vi "PositionReceiverAngleGoal.vi"(8 "error in (no error)":errorcluster, 9 "atacando contra":bool, 10 "Game":refnum<class "Game.lvclass">, 11 "PositionToReceivePassSkill in":refnum<class "PositionToReceivePassSkill.lvclass">) -> (0 "error out":errorcluster, 2 "theta final":dbl, 3 "PositionToReceivePassSkill out":refnum<class "PositionToReceivePassSkill.lvclass">)   [LabVIEW 2023, in "PositionToReceivePassSkill.lvclass"]
uses:
  PositionToReceivePassSkill.lvclass
  Game_class/Game.lvclass
  Game_class/Game.lvclass/Game.ctl
  Object_class/Object.lvclass/Object.ctl
  Team_class/Team.lvclass/Team.ctl
  Robot_class/roles.ctl
  Robot_class/Robot.lvclass/Robot.ctl
  Object_class/Read x.vi
  Object_class/Write x.vi
  Robot_class/Read role.vi
  Robot_class/Read id.vi
  Object_class/Read y.vi
  Game_class/Read BallRef.vi
  Game_class/Read EnemyRef.vi
  Game_class/Read FieldRef.vi
  Game_class/Read DefensiveTeam.vi
  Game_class/Read KeeperTeam.vi
  Team_class/Read RobotRef.vi
  Ally_class/Ally.lvclass
  Enemy_class/Enemy.lvclass
  Robot_class/Robot.lvclass
  Ball_class/Ball.lvclass
  Field_class/Field.lvclass
panel:
  in  "Array":dbl[](array[numeric])=[0.0, 0.0, 0.0, 0.0, 0.0, 0.0]
  in  "Contador 2":dbl
  in  "fim do intervalo":dbl=-1.57
  in  "inicio do intervalo":dbl=-1.57
  in  "tamanho do intervalo":dbl
  in  "valor de theta":dbl
  in  "RobôsParaAnalisar":dbl[][](array[numeric])=[[99999.0, 99999.0], [99999.0, 99999.0], [99999.0, 99999.0], [99999.0, 99999.0], [99999.0, 99999.0], [99999.0, 99999.0], [99999.0, 99999.0]]
  in  "Contador":dbl
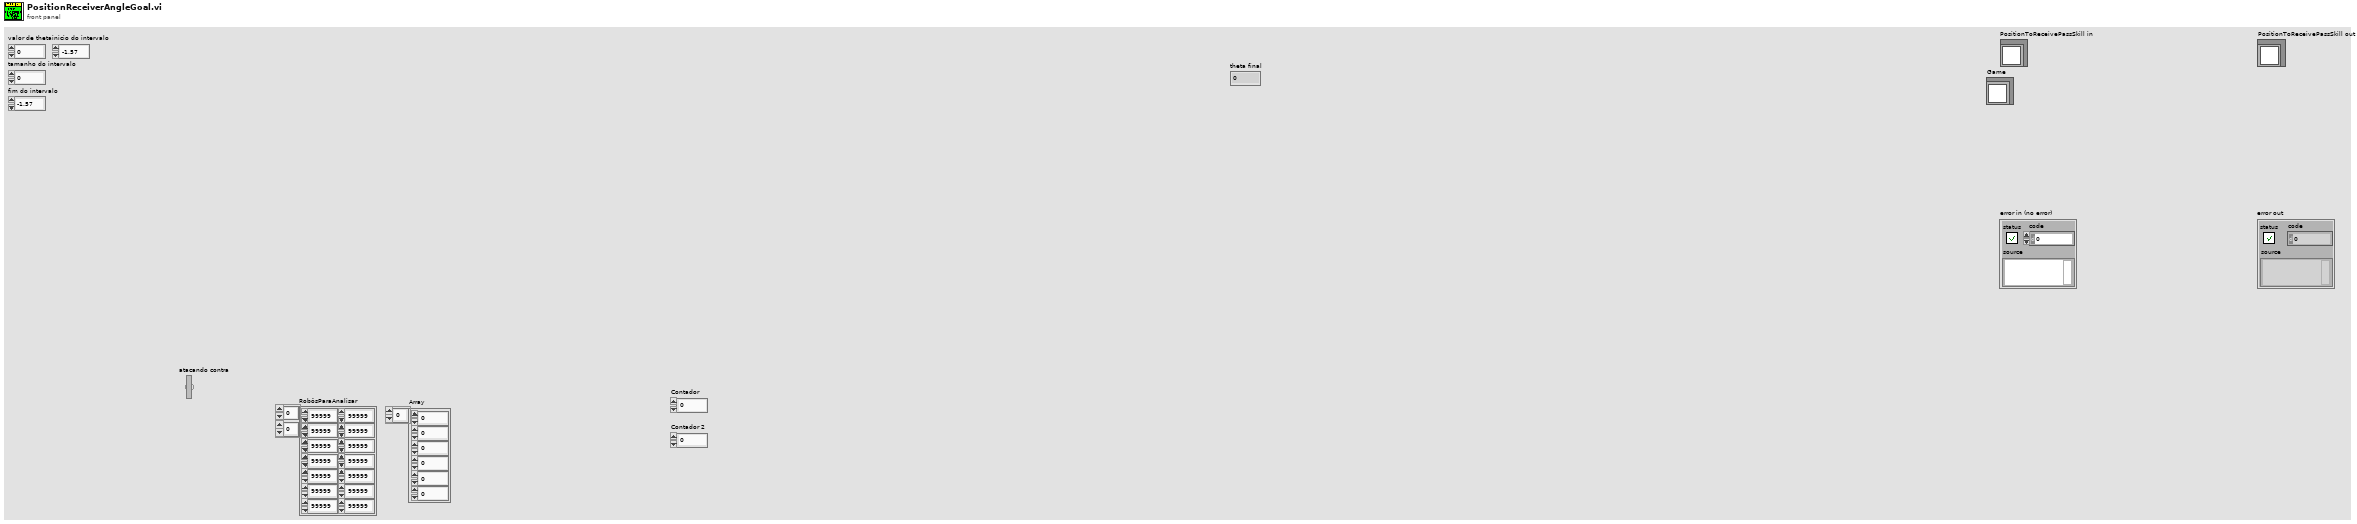
[diagram p1: front panel]
types:
  T1 = typedef "roles.ctl" = enum16{"BallChallengerAttackerVSS", "NormalAttackerVSS", "AttackerAimGoalVSS", "DefenderAreaVSS", "KeeperVSS", "Tabler", "TableFinalizer", "PrepareRollToPassRoller", "PrepareRollToPassReceiver", "SimplePassRoll", "SimplePassRollReceiver", "PenaltyDefense", "PreparePassReceiver 2", "PreparePassReceiver 1", "PassObserver", "Timeout", "Goto", "ZigZag", "None", "BallOutOfField", "DefenderArea", "Duelist", "AttackerStop", "FollowAttacker", "KeeperRole", "KickPenalty", "AttackerAimGoal", "AttackerBlock", "Marker", "Halt", "Shoot", "PassKicker", "PassReceiver", "TestRole", "PenaltyAttacker"}
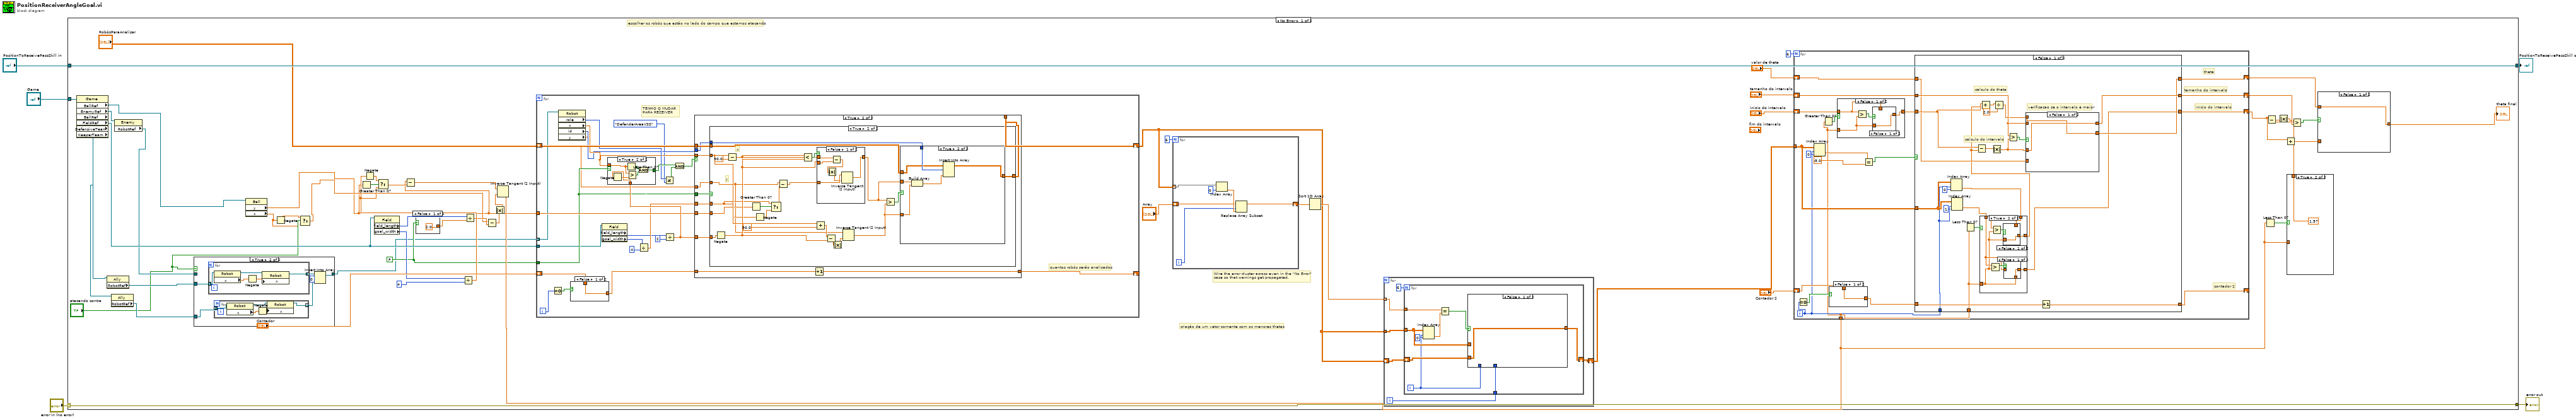
[diagram p0: block diagram]
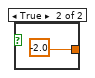
[diagram p4: hidden frame]
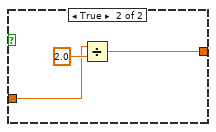
[diagram p5: hidden frame]
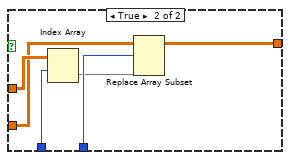
[diagram p6: hidden frame]
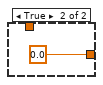
[diagram p9: hidden frame]
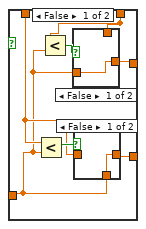
[diagram p10: hidden frame]
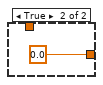
[diagram p17: hidden frame]
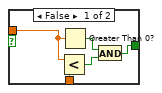
[diagram p18: hidden frame]
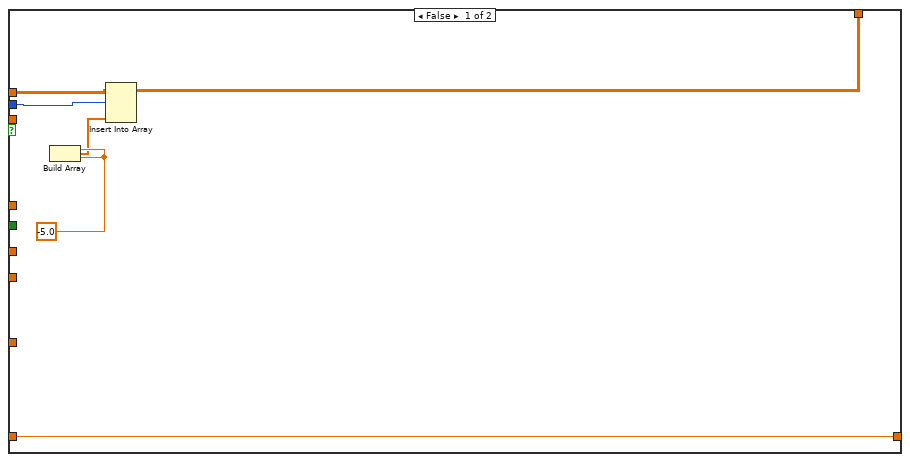
[diagram p19: hidden frame]
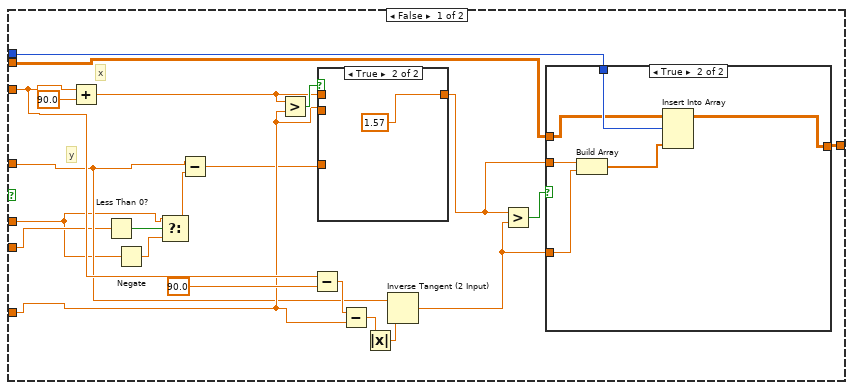
[diagram p20: hidden frame]
diagram:
  n1 = case shown="No Error" "error in (no error)" {
    selector: "error in (no error)" -> [w58 w333]
    tunnel: [w58 w333] -> w4
    tunnel: [w59 w332] -> w2
    tunnel: "PositionToReceivePassSkill in" -> [w59 w332]
    tunnel: "Game" -> [w23 _]
    frame No Error {
      w18 = FALSE
      # "criação de um vetor somente com os menores thetas"
      # "escolher os robôs que estão no lado do campo que estamos atacando"
      # "Wire the error cluster across even in the \"No Error\"\ncase so that warnings get propagated."
      n2 = property class="Game" props=["BallRef", "EnemyRef", "BallRef", "FieldRef", "DefensiveTeam", "KeeperTeam"](reference=w23) -> ("BallRef"=w9:refnum<class "Ball.lvclass">, "EnemyRef"=w22:refnum<class "Enemy.lvclass">, "FieldRef"=w21:refnum<class "Field.lvclass">, "DefensiveTeam"=w16:refnum<class "Ally.lvclass">, "KeeperTeam"=w11:refnum<class "Ally.lvclass">)  [unwired: 1 in, 3 out]
      n3 = property class="Ally"(reference=w16) -> ("RobotRef"=w14:refnum<class "Robot.lvclass">[])  [unwired: 1 in, 2 out]
      n4 = property class="Ally"(reference=w11) -> ("RobotRef"=w12:refnum<class "Robot.lvclass">[])  [unwired: 1 in, 2 out]
      n5 = property class="Enemy"(reference=w22) -> ("RobotRef"=w15:refnum<class "Robot.lvclass">[])  [unwired: 1 in, 2 out]
      n6 = case shown="True" "atacando contra" {
        tunnel: [w60 w61] -> w13
        tunnel: w15 -> [w60 _]
        tunnel: w14 -> [_ w66]
        tunnel: w12 -> [_ w65]
        frame False {
        }
        frame True {
          n7 = for {
            tunnel: [w74] -> w64 mode=indexing
            tunnel: w66 -> [w72] mode=indexing
            n8 = property class="Robot"(reference=w72) -> (reference out=w73:refnum<class "Robot.lvclass">, "x"=w76:dbl)  [unwired: 1 in, 1 out]
            n9 = Negate(x=w76) -> (-x=w75:dbl)
            n10 = property class="Robot"(reference=w73, "x"=w75) -> (reference out=w74:refnum<class "Robot.lvclass">)  [unwired: 1 in, 1 out]
          }
          n11 = for {
            tunnel: w65 -> [w71] mode=indexing
            tunnel: [w67] -> w63 mode=indexing
            n12 = property class="Robot"(reference=w71) -> (reference out=w68:refnum<class "Robot.lvclass">, "x"=w70:dbl)  [unwired: 1 in, 1 out]
            n13 = Negate(x=w70) -> (-x=w69:dbl)
            n14 = property class="Robot"(reference=w68, "x"=w69) -> (reference out=w67:refnum<class "Robot.lvclass">)  [unwired: 1 in, 1 out]
          }
          n15 = Insert Into Array(array=w64, index=0, new element=w63) -> (w61:refnum<class "Robot.lvclass">[])
        }
      }
      n16 = property class="Ball"(reference=w9) -> ("y"=w7:dbl, "x"=w6:dbl)  [unwired: 1 in, 2 out]
      n17 = Negate(x=w6) -> (-x=w8:dbl)
      n18 = Select(t=w8, s="atacando contra", f=w6) -> (s? t:f=w30:dbl)
      n19 = Greater Than 0?(x=w7) -> (x > 0?=w35:bool)
      n20 = property class="Field"(reference=w21) -> ("field_length"=w20:i32, "goal_width"=w19:i32)  [unwired: 1 in, 2 out]
      n21 = case shown="False" w18 {
        tunnel: [2.0 ("y") -2.0 ("y")] -> w28
        frame False {
        }
        frame True {
        }
      }
      n22 = Divide(x=w19, y=u32 4) -> (x/y=w33:dbl)
      n23 = Negate(x=w33) -> (-x=w34:dbl)
      n24 = Select(t=w34, s=w35, f=w33) -> (s? t:f=w32:dbl)
      n25 = Subtract(x=w7, y=w32) -> (x-y=w29:dbl)
      n26 = Divide(x=w20, y=w28) -> (x/y=w31:dbl)
      n27 = Subtract(x=w30, y=w31) -> (x-y=w25:dbl)
      n28 = Absolute Value(x=w25) -> (abs(x)=w24:dbl)
      n29 = Inverse Tangent (2 Input)(1:w24, 2:w29) -> (0:w26:dbl)
      n30 = for {
        tunnel: w13 -> [w202] mode=indexing
        tunnel: w18 -> [w207]
        shift-right: [w212] -> w46
        shift-left: "RobôsParaAnalisar" -> [w218]
        shift-right: [w213] -> _
        shift-left: "Contador" -> [w215]
        tunnel: w21 -> [w197]
        tunnel: w7 -> [w210]
        i -> [w216]
        # "TENHO Q MUDAR \nPARA RECEIVER"
        # "quantos robôs serão analisados"
        n31 = Equal To 0?(x=w216) -> (x = 0?=w217:bool)
        n32 = property class="Robot"(reference=w202) -> ("role"=w201:T1, "x"=w200:dbl, "id"=w199:i32, "y"=w198:dbl)  [unwired: 1 in, 2 out]
        n33 = case shown="False" w217 {
          tunnel: w215 -> [w219 _]
          tunnel: [w219 0.0] -> w214
          frame False {
          }
          frame True {
          }
        }
        n34 = property class="Field"(reference=w197) -> ("field_length"=w196:i32, "goal_width"=w195:i32)  [unwired: 1 in, 2 out]
        n35 = Divide(x=w195, y=u32 4) -> (x/y=w208:dbl)
        n36 = Not Equal?(x=w201, y=roles."DefenderAreaVSS") -> (x != y?=w204:bool)
        n37 = Divide(x=w196, y=u32 2) -> (x/y=w211:dbl)
        n38 = case shown="True" w207 {
          tunnel: w200 -> [w225 w226]
          tunnel: [w221 w231] -> w203
          tunnel: w211 -> [w224 w227]
          frame False {
            n39 = Less?(x=w225, y=w224) -> (x < y?=w222:bool)
            n40 = Greater Than 0?(x=w225) -> (x > 0?=w223:bool)
            n41 = And(x=w223, y=w222) -> (x .and. y?=w221:bool)
          }
          frame True {
            n42 = Negate(x=w227) -> (-x=w228:dbl)
            n43 = Less Than 0?(x=w226) -> (x < 0?=w230:bool)
            n44 = Greater?(x=w226, y=w228) -> (0:w229:bool)
            n45 = And(x=w230, y=w229) -> (x .and. y?=w231:bool)
          }
        }
        n46 = And(x=w203, y=w204) -> (x .and. y?=w205:bool)
        n47 = case shown="True" w205 {
          tunnel: w218 -> [w236 w243]
          tunnel: w199 -> [w235 w241]
          tunnel: w200 -> [_ w245]
          tunnel: w198 -> [_ w242]
          tunnel: w214 -> [w237 w247]
          tunnel: [w237 w248] -> w213
          tunnel: [w232 w240] -> w212
          tunnel: w207 -> [_ w246]
          tunnel: w211 -> [_ w244]
          tunnel: w210 -> [_ w239]
          tunnel: w208 -> [_ w238]
          frame False {
            w234 = -5.0 ("element")
            n48 = Build Array(w234, w234) -> (w233:dbl[])
            n49 = Insert Into Array(array=w236, index (row)=w235, new element=w233) -> (w232:dbl[][])  [unwired: 1 in]
          }
          frame True {
            n50 = case shown="True" w246 {
              tunnel: w245 -> [w260 w308]
              tunnel: w244 -> [w259 w311]
              tunnel: w243 -> [w261 w303]
              tunnel: w242 -> [w252 w292]
              tunnel: w241 -> [w262 w302]
              tunnel: [w258 w299] -> w240
              tunnel: w239 -> [w251 w296]
              tunnel: w238 -> [w250 w293]
              frame False {
                # "y"
                # "x"
                n51 = Add(x=w260, y=90.0) -> (x+y=w268:dbl)
                n52 = Less Than 0?(x=w251) -> (x < 0?=w255:bool)
                n53 = Negate(x=w250) -> (-x=w254:dbl)
                n54 = Select(t=w250, s=w255, f=w254) -> (s? t:f=w253:dbl)
                n55 = Subtract(x=w252, y=w253) -> (x-y=w249:dbl)
                n56 = Greater?(x=w268, y=w259) -> (0:w269:bool)
                n57 = Subtract(x=w260, y=90.0) -> (x-y=w266:dbl)
                n58 = case shown="True" w269 {
                  tunnel: w268 -> [w288 _]
                  tunnel: [w285 1.57] -> w264
                  tunnel: w259 -> [w287 _]
                  tunnel: w249 -> [w286 _]
                  frame False {
                    n59 = Subtract(x=w288, y=w287) -> (x-y=w284:dbl)
                    n60 = Absolute Value(x=w284) -> (abs(x)=w283:dbl)
                    n61 = Inverse Tangent (2 Input)(1:w283, 2:w286) -> (0:w285:dbl)
                  }
                  frame True {
                  }
                }
                n62 = Subtract(x=w266, y=w259) -> (x-y=w256:dbl)
                n63 = Absolute Value(x=w256) -> (abs(x)=w257:dbl)
                n64 = Inverse Tangent (2 Input)(1:w257, 2:w252) -> (0:w263:dbl)
                n65 = Greater?(x=w264, y=w263) -> (0:w265:bool)
                n66 = case shown="True" w265 {
                  tunnel: w261 -> [w273 w279]
                  tunnel: w262 -> [w275 w282]
                  tunnel: w264 -> [w272 w280]
                  tunnel: w263 -> [w274 w278]
                  tunnel: [w271 w277] -> w258
                  frame False {
                    n67 = Build Array(w274, w272) -> (w276:dbl[])
                    n68 = Insert Into Array(array=w273, index (row)=w275, new element=w276) -> (w271:dbl[][])  [unwired: 1 in]
                  }
                  frame True {
                    n69 = Build Array(w280, w278) -> (w281:dbl[])
                    n70 = Insert Into Array(array=w279, index (row)=w282, new element=w281) -> (w277:dbl[][])  [unwired: 1 in]
                  }
                }
              }
              frame True {
                # "y"
                # "x"
                n71 = Negate(x=w311) -> (-x=w305:dbl)
                n72 = Subtract(x=w308, y=90.0) -> (x-y=w309:dbl)
                n73 = Greater Than 0?(x=w296) -> (x > 0?=w295:bool)
                n74 = Negate(x=w293) -> (-x=w294:dbl)
                n75 = Select(t=w293, s=w295, f=w294) -> (s? t:f=w291:dbl)
                n76 = Subtract(x=w292, y=w291) -> (x-y=w290:dbl)
                n77 = Less?(x=w309, y=w305) -> (x < y?=w310:bool)
                n78 = Add(x=w308, y=90.0) -> (x+y=w306:dbl)
                n79 = case shown="False" w310 {
                  tunnel: w309 -> [w330 _]
                  tunnel: [w327 1.57] -> w301
                  tunnel: w305 -> [w329 _]
                  tunnel: w290 -> [w328 _]
                  frame False {
                    n80 = Subtract(x=w330, y=w329) -> (x-y=w325:dbl)
                    n81 = Absolute Value(x=w325) -> (abs(x)=w326:dbl)
                    n82 = Inverse Tangent (2 Input)(1:w326, 2:w328) -> (0:w327:dbl)
                  }
                  frame True {
                  }
                }
                n83 = Subtract(x=w306, y=w305) -> (x-y=w297:dbl)
                n84 = Absolute Value(x=w297) -> (abs(x)=w298:dbl)
                n85 = Inverse Tangent (2 Input)(1:w298, 2:w292) -> (0:w300:dbl)
                n86 = Greater?(x=w301, y=w300) -> (0:w304:bool)
                n87 = case shown="True" w304 {
                  tunnel: w303 -> [w315 w321]
                  tunnel: w302 -> [w317 w324]
                  tunnel: w301 -> [w314 w322]
                  tunnel: w300 -> [w316 w320]
                  tunnel: [w313 w319] -> w299
                  frame False {
                    n88 = Build Array(w316, w314) -> (w318:dbl[])
                    n89 = Insert Into Array(array=w315, index (row)=w317, new element=w318) -> (w313:dbl[][])  [unwired: 1 in]
                  }
                  frame True {
                    n90 = Build Array(w322, w320) -> (w323:dbl[])
                    n91 = Insert Into Array(array=w321, index (row)=w324, new element=w323) -> (w319:dbl[][])  [unwired: 1 in]
                  }
                }
              }
            }
            n92 = Increment(x=w247) -> (x+1=w248:dbl)
          }
        }
      }
      n93 = for {
        N: 6 -> [_]
        tunnel: w46 -> [w112] mode=indexing
        shift-right: [w107] -> w48
        shift-left: "Array" -> [w108]
        i -> [w109]
        n94 = Index Array(array=w112, index=0) -> (element=w110:dbl)
        n95 = Replace Array Subset(array=w108, new element=w110, index=w109) -> (w107:dbl[])
      }
      n96 = Sort 1D Array(array=w48) -> (sorted array=w47:dbl[])
      n97 = for {
        tunnel: w47 -> [w87] mode=indexing
        tunnel: w46 -> [w89]
        shift-right: [w85] -> w45
        shift-left: w46 -> [w88]
        i -> [w86]
        n98 = for {
          N: 6 -> [_]
          tunnel: w89 -> [w95]
          shift-right: [w91] -> w85
          shift-left: w88 -> [w94]
          tunnel: w87 -> [w97]
          tunnel: w86 -> [w92]
          i -> [w93]
          n99 = Index Array(array=w95, index (row)=w93, index (col)=0 ("disabled index (col)")) -> (element=w98:dbl)
          n100 = Equal?(x=w97, y=w98) -> (x = y?=w96:bool)
          n101 = case shown="False" w96 {
            tunnel: w95 -> [_ w106]
            tunnel: w94 -> [w100 w102]
            tunnel: w93 -> [_ w105]
            tunnel: w92 -> [_ w104]
            tunnel: [w100 w101] -> w91
            frame False {
            }
            frame True {
              n102 = Index Array(array=w106, index (row)=w105) -> (element=w103:dbl[])  [unwired: 1 in]
              n103 = Replace Array Subset(array=w102, new element=w103, index (row)=w104) -> (w101:dbl[][])  [unwired: 1 in]
            }
          }
        }
      }
      n104 = for {
        N: 6 -> [_]
        tunnel: w45 -> [w120]
        shift-right: [w128] -> w42
        shift-left: "valor de theta" -> [w129]
        shift-right: [w126] -> w44
        shift-left: "tamanho do intervalo" -> [w127]
        shift-right: [w125] -> w39
        shift-left: "inicio do intervalo" -> [w114]
        shift-right: [w121] -> _
        shift-left: "Contador 2" -> [w123]
        tunnel: w26 -> [w113]
        i -> [w119]
        # "contador 2"
        # "inicio do intervalo"
        # "tamanho do intervalo"
        # "theta"
        n105 = Equal To 0?(x=w119) -> (x = 0?=w124:bool)
        n106 = Index Array(array=w120, index (row)=w119, index (col)=0 ("disabled index (col)")) -> (element=w118:dbl)
        n107 = Greater Than 0?(x=w113) -> (x > 0?=w116:bool)
        n108 = case shown="False" w124 {
          tunnel: w123 -> [w139 _]
          tunnel: [w139 0.0] -> w122
          frame False {
          }
          frame True {
          }
        }
        n109 = case shown="False" w116 {
          tunnel: [w134 w138] -> w115
          tunnel: w114 -> [w133 w138]
          tunnel: w113 -> [w132 _]
          frame False {
            n110 = Greater?(x=w133, y=w132) -> (0:w135:bool)
            n111 = case shown="False" w135 {
              tunnel: [w136 w137] -> w134
              tunnel: w133 -> [_ w137]
              tunnel: w132 -> [w136 _]
              frame False {
              }
              frame True {
              }
            }
          }
          frame True {
          }
        }
        n112 = Equal?(x=w118, y=-5.0) -> (x = y?=w117:bool)
        n113 = case shown="False" w117 {
          tunnel: w129 -> [w147 w193]
          tunnel: [w148 w193] -> w128
          tunnel: w127 -> [w152 w192]
          tunnel: [w151 w192] -> w126
          tunnel: w115 -> [w163 w191]
          tunnel: [w141 w191] -> w125
          tunnel: w122 -> [w161 w190]
          tunnel: [w162 w190] -> w121
          tunnel: w120 -> [w160 _]
          tunnel: w119 -> [w159 _]
          tunnel: w113 -> [w145 _]
          frame False {
            # "calculo do theta"
            # "calculo do intervalo"
            # "verificacao se o intervalo é maior"
            n114 = Index Array(array=w160, index (row)=w159, index (col)=0 ("disabled index (col)")) -> (element=w144:dbl)
            n115 = Index Array(array=w160, index (row)=w159, index (col)=1 ("disabled index (col)")) -> (element=w142:dbl)
            n116 = Less Than 0?(x=w145) -> (x < 0?=w146:bool)
            n117 = case shown="True" w146 {
              tunnel: w142 -> [w168 w177]
              tunnel: w144 -> [w164 w179]
              tunnel: w145 -> [w167 w175]
              tunnel: [w166 w180] -> w143
              tunnel: [w165 w176] -> w141
              frame False {
                n118 = Less?(x=w168, y=w167) -> (x < y?=w170:bool)
                n119 = Less?(x=w164, y=w167) -> (x < y?=w169:bool)
                n120 = case shown="False" w169 {
                  tunnel: [w173 w174] -> w166
                  tunnel: w164 -> [_ w174]
                  tunnel: w167 -> [w173 _]
                  frame False {
                  }
                  frame True {
                  }
                }
                n121 = case shown="False" w170 {
                  tunnel: w168 -> [_ w172]
                  tunnel: [w171 w172] -> w165
                  tunnel: w167 -> [w171 _]
                  frame False {
                  }
                  frame True {
                  }
                }
              }
              frame True {
                n122 = Greater?(x=w177, y=w175) -> (0:w178:bool)
                n123 = Greater?(x=w179, y=w175) -> (0:w181:bool)
                n124 = case shown="False" w181 {
                  tunnel: [w184 w185] -> w180
                  tunnel: w179 -> [_ w185]
                  tunnel: w175 -> [w184 _]
                  frame False {
                  }
                  frame True {
                  }
                }
                n125 = case shown="False" w178 {
                  tunnel: w177 -> [_ w183]
                  tunnel: [w182 w183] -> w176
                  tunnel: w175 -> [w182 _]
                  frame False {
                  }
                  frame True {
                  }
                }
              }
            }
            n126 = Subtract(x=w163, y=w143) -> (x-y=w156:dbl)
            n127 = Add(x=w163, y=w143) -> (x+y=w155:dbl)
            n128 = Absolute Value(x=w156) -> (abs(x)=w150:dbl)
            n129 = Divide(x=w155, y=2.0) -> (x/y=w149:dbl)
            n130 = Greater?(x=w152, y=w150) -> (0:w153:bool)
            n131 = case shown="False" w153 {
              tunnel: w152 -> [_ w189]
              tunnel: [w187 w189] -> w151
              tunnel: w150 -> [w187 _]
              tunnel: w147 -> [_ w188]
              tunnel: w149 -> [w186 _]
              tunnel: [w186 w188] -> w148
              frame False {
              }
              frame True {
              }
            }
            n132 = Increment(x=w161) -> (x+1=w162:dbl)
          }
          frame True {
          }
        }
      }
      n133 = Less Than 0?(x=w26) -> (x < 0?=w27:bool)
      n134 = case shown="True" w27 {
        tunnel: [w77 1.57 ("y")] -> w38
        tunnel: w26 -> [w77 _]
        frame False {
        }
        frame True {
        }
      }
      n135 = Subtract(x=w39, y=w38) -> (x-y=w41:dbl)
      n136 = Absolute Value(x=w41) -> (abs(x)=w40:dbl)
      n137 = Add(x=w39, y=w38) -> (x+y=w37:dbl)
      n138 = Greater?(x=w40, y=w44) -> (0:w43:bool)
      n139 = case shown="False" w43 {
        tunnel: [w81 w83] -> w17
        tunnel: w42 -> [w81 _]
        tunnel: w37 -> [_ w82]
        frame False {
        }
        frame True {
          n140 = Divide(x=w82, y=2.0) -> (x/y=w83:dbl)
        }
      }
      "theta final" <- w17
    }
    frame Error {
    }
  }
  "error out" <- w4
  "PositionToReceivePassSkill out" <- w2
